vi "getMessageEndChar.vi"(8 "error in (no error)":errorcluster, 10 "messageEnd":string, 11 "TCPClient in":refnum<class "TCPClient.lvclass">) -> (0 "error out":errorcluster, 2 "message":string, 3 "TCPClient out":refnum<class "TCPClient.lvclass">)   [LabVIEW 2016, in "tcp.lvlib" / "TCPClient.lvclass"]
uses:
  TCPClient.lvclass
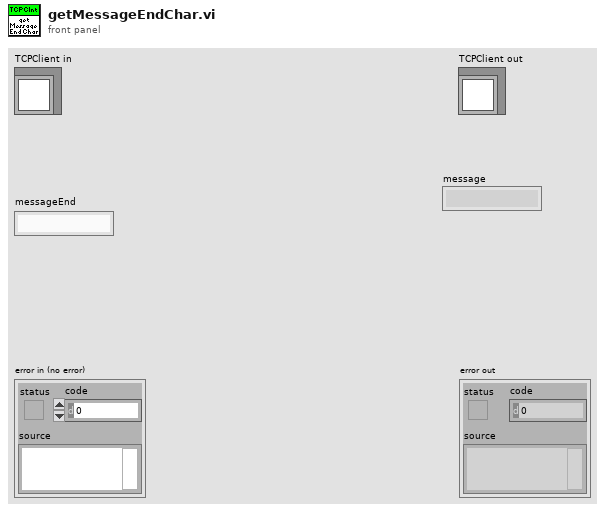
[diagram p1: front panel]
types:
  T1 = enum16{"Standard", "Buffered", "CRLF", "Immediate"}
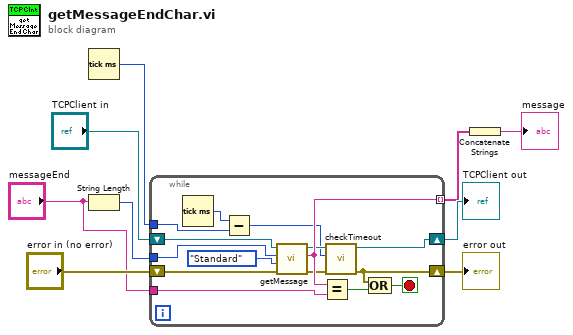
[diagram p0: block diagram]
diagram:
  n1 = Tick Count (ms)() -> (millisecond timer value=w1:u32)
  n2 = String Length(string="messageEnd") -> (length=w2:i32)
  n3 = while {
    shift-right: [w11] -> w8
    shift-left: "TCPClient in" -> [w24]
    shift-right: [w13] -> w6
    shift-left: "error in (no error)" -> [w23]
    tunnel: [w20] -> w5 mode=indexing
    tunnel: "messageEnd" -> [w19]
    tunnel: w2 -> [w18]
    tunnel: w1 -> [w16]
    stop <- w21 stop-if-true
    n4 = Tick Count (ms)() -> (millisecond timer value=w15:u32)
    n5 = Subtract(x=w15, y=w16) -> (x-y=w10:u32)
    n6 = call-dynamic "getMessage.vi"("error in (no error)"=w23, "mode (standard)"=T1."Standard", "bytes to read"=w18, "TCPClient in"=w24) -> ("error out"=w14:errorcluster, "message"=w20:string, "TCPClient out"=w12:refnum<class "TCPClient.lvclass">)  [unwired: 5 in]
    n7 = Equal?(x=w20, y=w19) -> (x = y?=w17:bool)
    n8 = call "checkTimeout.vi"("error in (no error)"=w14, "executionTime"=w10, "TCPClient in"=w12) -> ("error out"=w13:errorcluster, "TCPClient out"=w11:refnum<class "TCPClient.lvclass">)  [unwired: 7 in]
    n9 = Compound Arithmetic op=OR(w13, w17) -> (w21:bool)
  }
  "error out" <- w6
  "TCPClient out" <- w8
  n10 = Concatenate Strings(w5) -> (→"message":string)
